vi "String from C-string pointer.vi"(8 "error in (no error)":errorcluster, 9 "Bytes to copy":i32, 10 "Pointer":i64) -> (0 "error out":errorcluster, 3 "string":string)   [LabVIEW 2023, in "SQLiteSupport.lvlib"]
uses:
  SQLiteSupport.lvlib
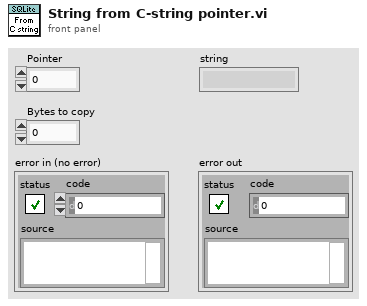
[diagram p1: front panel]
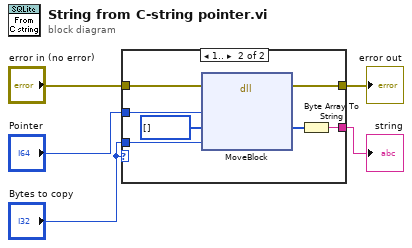
[diagram p0: block diagram]
diagram:
  n1 = case shown="1.." "Bytes to copy" {
    tunnel: "Bytes to copy" -> [_ w13]
    tunnel: "Pointer" -> [_ w12]
    tunnel: [_ w11] -> w4
    tunnel: [w6 w9] -> w3
    tunnel: "error in (no error)" -> [w6 w7]
    frame ..0 {
    }
    frame 1.. {
      n2 = dll-call lib="LabVIEW" fn="MoveBlock"(error in=w7, "source"=w12, "destination"=u8[] [], "size"=w13) -> (error out=w9:errorcluster, "destination"=w8:u8[])  [unwired: 5 in, 1 out]
      n3 = Byte Array To String(unsigned byte array=w8) -> (string=w11:string)
    }
  }
  "string" <- w4
  "error out" <- w3
